vi "Loss测量.vi"(8 "error in (no error)":errorcluster, 9 "Freq":dbl[](array[numeric]), 11 "VISA resource name":refnum<visa-resource-name>) -> (0 "S22":dbl[](array[numeric]), 1 "S21":dbl[](array[numeric]), 2 "S12":dbl[](array[numeric]), 3 "S11":dbl[](array[numeric]), 4 "error out":errorcluster, 5 "freq":dbl[](array[numeric]))   [LabVIEW 2011]
uses:
  Agilent ENA Series/Agilent ENA Series.lvlib
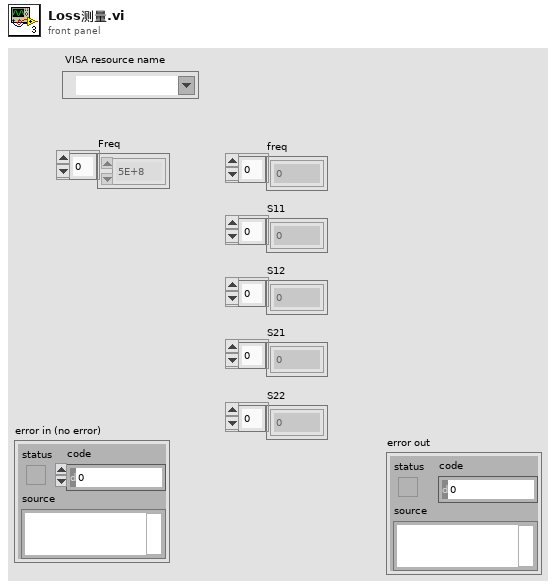
[diagram p1: front panel]
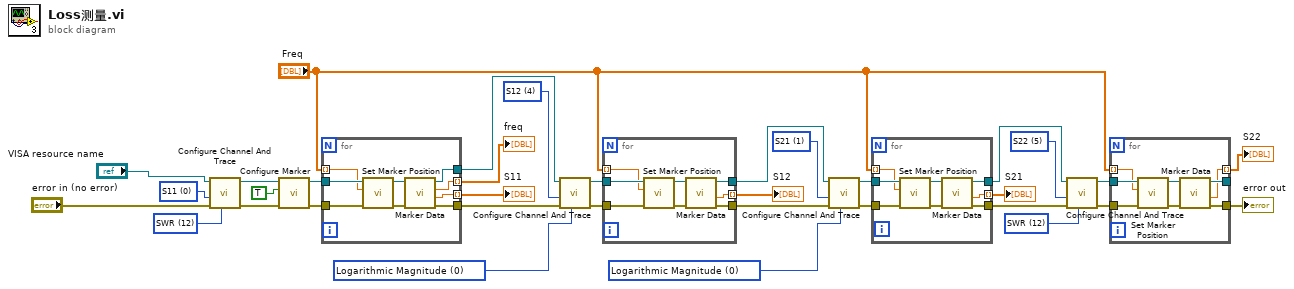
[diagram p0: block diagram]
diagram:
  w3 = u16 12 items=["Logarithmic Magnitude", "Phase", "Group Delay", "Smith Chart  Linear (Lin/Phase)", "Smith Chart  Logarithmic (Log/Phase)", "Smith Chart  Complex (Real/Imag)", "Smith Chart  Impedance (R+jX)", "Smith Chart  Admittance (G+jB)", "Polar Format (Linear)", "Polar Format (Logarithmic)", "Polar Format (Re/Im)", "Linear Magnitude", "SWR", "Real", "Imaginary", "Epanded Phase", "Positive Phase"] ("Data Format (0: Logarithmic Magnitude)")
  w9 = u16 5 items=["S11", "S21", "S31", "S41", "S12", "S22", "S32", "S42", "S13", "S23", "S33", "S43", "S14", "S24", "S34", "S44", "A", "B", "C", "D", "R1", "R2", "R3", "R4", "AUX1", "AUX2", "TR", "T", "R"] ("Measurement Parameters (0: S11)")
  w13 = u16 0 items=["Logarithmic Magnitude", "Phase", "Group Delay", "Smith Chart  Linear (Lin/Phase)", "Smith Chart  Logarithmic (Log/Phase)", "Smith Chart  Complex (Real/Imag)", "Smith Chart  Impedance (R+jX)", "Smith Chart  Admittance (G+jB)", "Polar Format (Linear)", "Polar Format (Logarithmic)", "Polar Format (Re/Im)", "Linear Magnitude", "SWR", "Real", "Imaginary", "Epanded Phase", "Positive Phase"] ("Data Format (0: Logarithmic Magnitude)")
  w12 = u16 1 items=["S11", "S21", "S31", "S41", "S12", "S22", "S32", "S42", "S13", "S23", "S33", "S43", "S14", "S24", "S34", "S44", "A", "B", "C", "D", "R1", "R2", "R3", "R4", "AUX1", "AUX2", "TR", "T", "R"] ("Measurement Parameters (0: S11)")
  w22 = u16 0 items=["Logarithmic Magnitude", "Phase", "Group Delay", "Smith Chart  Linear (Lin/Phase)", "Smith Chart  Logarithmic (Log/Phase)", "Smith Chart  Complex (Real/Imag)", "Smith Chart  Impedance (R+jX)", "Smith Chart  Admittance (G+jB)", "Polar Format (Linear)", "Polar Format (Logarithmic)", "Polar Format (Re/Im)", "Linear Magnitude", "SWR", "Real", "Imaginary", "Epanded Phase", "Positive Phase"] ("Data Format (0: Logarithmic Magnitude)")
  w23 = u16 4 items=["S11", "S21", "S31", "S41", "S12", "S22", "S32", "S42", "S13", "S23", "S33", "S43", "S14", "S24", "S34", "S44", "A", "B", "C", "D", "R1", "R2", "R3", "R4", "AUX1", "AUX2", "TR", "T", "R"] ("Measurement Parameters (0: S11)")
  w31 = u16 12 items=["Logarithmic Magnitude", "Phase", "Group Delay", "Smith Chart  Linear (Lin/Phase)", "Smith Chart  Logarithmic (Log/Phase)", "Smith Chart  Complex (Real/Imag)", "Smith Chart  Impedance (R+jX)", "Smith Chart  Admittance (G+jB)", "Polar Format (Linear)", "Polar Format (Logarithmic)", "Polar Format (Re/Im)", "Linear Magnitude", "SWR", "Real", "Imaginary", "Epanded Phase", "Positive Phase"] ("Data Format (0: Logarithmic Magnitude)")
  w32 = u16 0 items=["S11", "S21", "S31", "S41", "S12", "S22", "S32", "S42", "S13", "S23", "S33", "S43", "S14", "S24", "S34", "S44", "A", "B", "C", "D", "R1", "R2", "R3", "R4", "AUX1", "AUX2", "TR", "T", "R"] ("Measurement Parameters (0: S11)")
  n1 = call "Configure Channel And Trace.vi"("Data Format (0: Logarithmic Magnitude)"=w31, "error in (no error)"="error in (no error)", "Measurement Parameters (0: S11)"=w32, "VISA resource name"="VISA resource name") -> ("error out"=w29:errorcluster, "VISA resource name out"=w30:refnum<visa-resource-name>)  [unwired: 6 in]
  n2 = call "Configure Marker.vi"("error in (no error)"=w29, "Marker State (F: Disabled)"=TRUE, "VISA resource name"=w30) -> ("error out"=w26:errorcluster, "VISA resource name out"=w27:refnum<visa-resource-name>)  [unwired: 7 in]
  n3 = for {
    tunnel: w27 -> [w43]
    tunnel: w26 -> [w42]
    tunnel: [w39] -> w21
    tunnel: [w38] -> w20
    tunnel: "Freq" -> [w37] mode=indexing
    tunnel: [w36] -> w25 mode=indexing
    tunnel: [w35] -> w24 mode=indexing
    n4 = call "Set Marker Position.vi"("error in (no error)"=w42, "X Value (0.0)"=w37, "VISA resource name"=w43) -> ("error out"=w40:errorcluster, "VISA resource name out"=w41:refnum<visa-resource-name>)  [unwired: 7 in]
    n5 = call "Marker Data.vi"("error in (no error)"=w40, "VISA resource name"=w41) -> ("error out"=w38:errorcluster, "Y Real Value"=w35:dbl, "X Value"=w36:dbl, "VISA resource name out"=w39:refnum<visa-resource-name>)  [unwired: 5 in, 1 out]
  }
  "freq" <- w25
  "S11" <- w24
  n6 = call "Configure Channel And Trace.vi"("Data Format (0: Logarithmic Magnitude)"=w22, "error in (no error)"=w20, "Measurement Parameters (0: S11)"=w23, "VISA resource name"=w21) -> ("error out"=w18:errorcluster, "VISA resource name out"=w19:refnum<visa-resource-name>)  [unwired: 6 in]
  n7 = for {
    tunnel: w19 -> [w51]
    tunnel: w18 -> [w50]
    tunnel: [w47] -> w11
    tunnel: [w46] -> w10
    tunnel: "Freq" -> [w45] mode=indexing
    tunnel: [w44] -> w17 mode=indexing
    n8 = call "Set Marker Position.vi"("error in (no error)"=w50, "X Value (0.0)"=w45, "VISA resource name"=w51) -> ("error out"=w48:errorcluster, "VISA resource name out"=w49:refnum<visa-resource-name>)  [unwired: 7 in]
    n9 = call "Marker Data.vi"("error in (no error)"=w48, "VISA resource name"=w49) -> ("error out"=w46:errorcluster, "Y Real Value"=w44:dbl, "VISA resource name out"=w47:refnum<visa-resource-name>)  [unwired: 5 in, 2 out]
  }
  "S12" <- w17
  n10 = call "Configure Channel And Trace.vi"("Data Format (0: Logarithmic Magnitude)"=w13, "error in (no error)"=w10, "Measurement Parameters (0: S11)"=w12, "VISA resource name"=w11) -> ("error out"=w15:errorcluster, "VISA resource name out"=w14:refnum<visa-resource-name>)  [unwired: 6 in]
  n11 = for {
    tunnel: w14 -> [w59]
    tunnel: w15 -> [w58]
    tunnel: [w55] -> w5
    tunnel: [w54] -> w4
    tunnel: "Freq" -> [w53] mode=indexing
    tunnel: [w52] -> w16 mode=indexing
    n12 = call "Set Marker Position.vi"("error in (no error)"=w58, "X Value (0.0)"=w53, "VISA resource name"=w59) -> ("error out"=w56:errorcluster, "VISA resource name out"=w57:refnum<visa-resource-name>)  [unwired: 7 in]
    n13 = call "Marker Data.vi"("error in (no error)"=w56, "VISA resource name"=w57) -> ("error out"=w54:errorcluster, "Y Real Value"=w52:dbl, "VISA resource name out"=w55:refnum<visa-resource-name>)  [unwired: 5 in, 2 out]
  }
  "S21" <- w16
  n14 = call "Configure Channel And Trace.vi"("Data Format (0: Logarithmic Magnitude)"=w3, "error in (no error)"=w4, "Measurement Parameters (0: S11)"=w9, "VISA resource name"=w5) -> ("error out"=w7:errorcluster, "VISA resource name out"=w8:refnum<visa-resource-name>)  [unwired: 6 in]
  n15 = for {
    tunnel: w8 -> [w67]
    tunnel: w7 -> [w66]
    tunnel: [w63] -> _
    tunnel: [w62] -> w1
    tunnel: "Freq" -> [w61] mode=indexing
    tunnel: [w60] -> w6 mode=indexing
    n16 = call "Set Marker Position.vi"("error in (no error)"=w66, "X Value (0.0)"=w61, "VISA resource name"=w67) -> ("error out"=w64:errorcluster, "VISA resource name out"=w65:refnum<visa-resource-name>)  [unwired: 7 in]
    n17 = call "Marker Data.vi"("error in (no error)"=w64, "VISA resource name"=w65) -> ("error out"=w62:errorcluster, "Y Real Value"=w60:dbl, "VISA resource name out"=w63:refnum<visa-resource-name>)  [unwired: 5 in, 2 out]
  }
  "S22" <- w6
  "error out" <- w1
